vi "PC_Pub_imgFile init.vi"(8 "error in (no error)":errorcluster, 11 "imgFile in":refnum<class "PC_Pub_imgFile.lvclass">) -> (0 "error out":errorcluster, 3 "imgFile out":refnum<class "PC_Pub_imgFile.lvclass">)   [LabVIEW 2018, in "PC_Pub_imgFile.lvclass"]
uses:
  PC_Pub_imgFile.lvclass
  PC_Pub_imgFile.lvclass/PC_Pub_imgFile.ctl
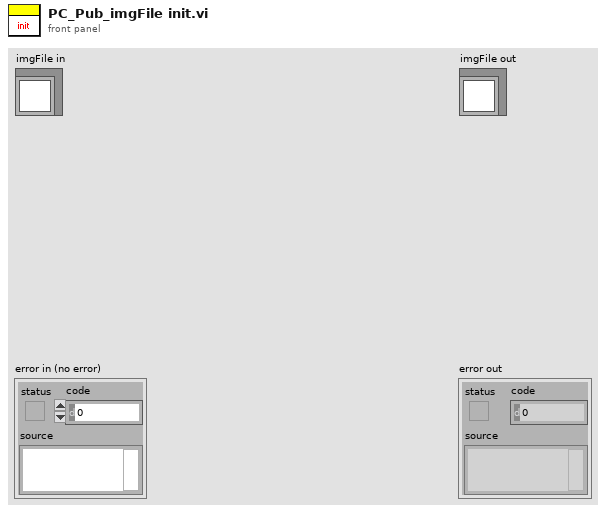
[diagram p1: front panel]
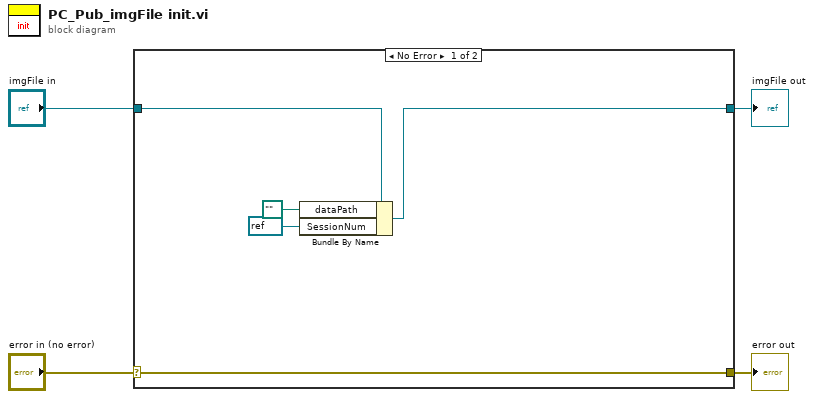
[diagram p0: block diagram]
diagram:
  n1 = case shown="No Error" "error in (no error)" {
    selector: "error in (no error)" -> [w9 w11]
    tunnel: [w9 w11] -> w3
    tunnel: [w5 w10] -> w1
    tunnel: "imgFile in" -> [w8 w10]
    frame No Error {
      n2 = Bundle By Name(cluster=w8, "dataPath"=path "", "SessionNum"=refnum<k21> refnum) -> (w5:refnum<class "PC_Pub_imgFile.lvclass">)
    }
    frame Error {
    }
  }
  "error out" <- w3
  "imgFile out" <- w1
